vi "Get Request Type.vi"(8 "error in (no error)":errorcluster, 11 "TriggerHotkeyByKeySequence in":refnum<class "TriggerHotkeyByKeySequence.lvclass">) -> (0 "error out":errorcluster, 2 "Request Type":string, 3 "TriggerHotkeyByKeySequence out":refnum<class "TriggerHotkeyByKeySequence.lvclass">)   [LabVIEW 2022 SP3, in "obs-websocket-lv.lvlib" / "TriggerHotkeyByKeySequence.lvclass"]
uses:
  TriggerHotkeyByKeySequence.lvclass
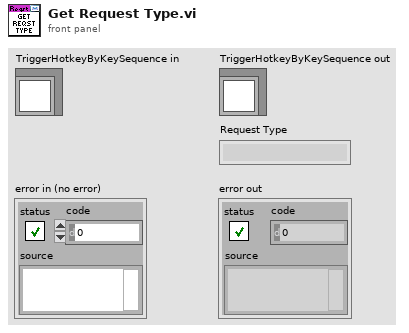
[diagram p1: front panel]
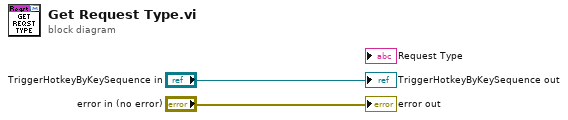
[diagram p0: block diagram]
diagram:
  "error out" <- "error in (no error)"
  "TriggerHotkeyByKeySequence out" <- "TriggerHotkeyByKeySequence in"
